vi "Potting Parameters.vi"(7 "Get/Set":enum16{"Get", "Set"}(ring), 8 "error in (no error)":errorcluster, 9 "Encapsulant":string, 10 "Potting Parameters in":T1, 11 "FlexWorktable in":refnum<class "FlexWorktable.lvclass">) -> (0 "error out":errorcluster, 2 "Potting Parameters out":T1, 3 "FlexWorktable out":refnum<class "FlexWorktable.lvclass">)   [LabVIEW 2017, in "FlexWorktable.lvclass"]
uses:
  FlexWorktable.lvclass
  Potting Parameters.ctl
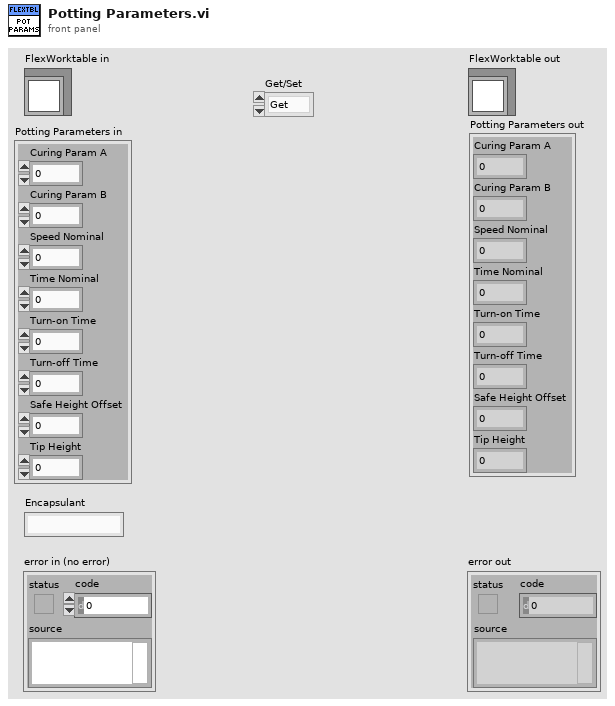
[diagram p1: front panel]
types:
  T1 = typedef "FlexWorktable.lvclass/Potting Parameters.ctl" = cluster{"Curing Param A":dbl, "Curing Param B":dbl, "Speed Nominal":dbl, "Time Nominal":dbl, "Turn-on Time":dbl, "Turn-off Time":dbl, "Safe Height Offset":dbl, "Tip Height":dbl}
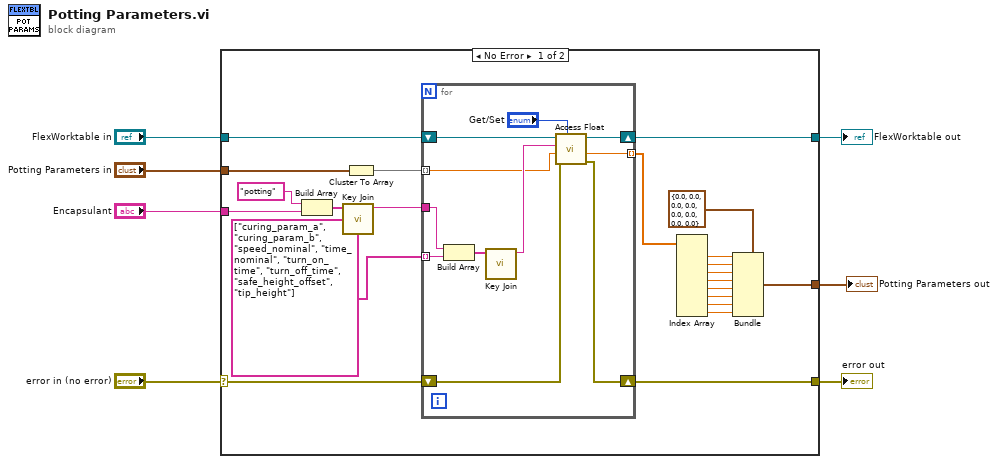
[diagram p0: block diagram]
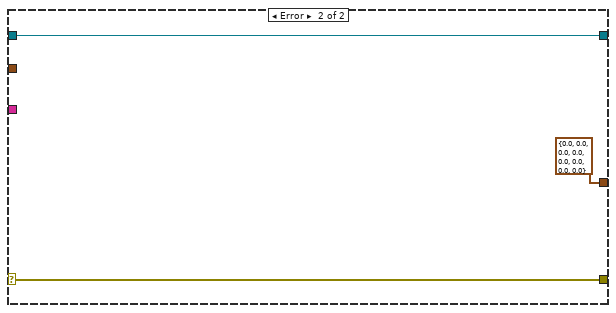
[diagram p2: hidden frame]
diagram:
  n1 = case shown="No Error" "error in (no error)" {
    selector: "error in (no error)" -> [w21 w43]
    tunnel: [w20 w43] -> w6
    tunnel: [w19 w42] -> w4
    tunnel: "FlexWorktable in" -> [w22 w42]
    tunnel: "Potting Parameters in" -> [w26 _]
    tunnel: "Encapsulant" -> [w27 _]
    tunnel: [w8 T1 {"Curing Param A"=0.0, "Curing Param B"=0.0, "Speed Nominal"=0.0, "Time Nominal"=0.0, "Turn-on Time"=0.0, "Turn-off Time"=0.0, "Safe Height Offset"=0.0, "Tip Height"=0.0} ("Potting Parameters in")] -> w1
    frame No Error {
      n2 = Build Array("potting", w27) -> (w29:string[])
      n3 = call "Key Join.vi"("Key Elements"=w29) -> ("Key"=w23:string)  [unwired: 10 in]
      n4 = Cluster To Array(cluster=w26) -> (array=w25:dbl[])
      n5 = for {
        tunnel: w25 -> [w34] mode=indexing
        tunnel: string[] ["curing_param_a", "curing_param_b", "speed_nominal", "time_nominal", "turn_on_time", "turn_off_time", "safe_height_offset", "tip_height"] -> [w39] mode=indexing
        tunnel: w23 -> [w40]
        shift-right: [w32] -> w20
        shift-left: w21 -> [w33]
        tunnel: [w31] -> w18 mode=indexing
        shift-right: [w30] -> w19
        shift-left: w22 -> [w35]
        n6 = Build Array(w40, w39) -> (w38:string[])
        n7 = call "Key Join.vi"("Key Elements"=w38) -> ("Key"=w37:string)  [unwired: 10 in]
        n8 = call-dynamic "Access Float.vi"("Get/Set"="Get/Set", "error in (no error)"=w33, "Value in"=w34, "Key"=w37, "FlexWorktable in"=w35) -> ("error out"=w32:errorcluster, "Value out"=w31:dbl, "FlexWorktable out"=w30:refnum<class "FlexWorktable.lvclass">)  [unwired: 4 in]
      }
      n9 = Index Array(array=w18) -> (element #1=w16:dbl, element #2=w15:dbl, element #3=w14:dbl, element #4=w13:dbl, element #5=w12:dbl, element #6=w11:dbl, element #7=w10:dbl, element #8=w9:dbl)  [unwired: 8 in]
      n10 = Bundle(cluster=T1 {"Curing Param A"=0.0, "Curing Param B"=0.0, "Speed Nominal"=0.0, "Time Nominal"=0.0, "Turn-on Time"=0.0, "Turn-off Time"=0.0, "Safe Height Offset"=0.0, "Tip Height"=0.0} ("Potting Parameters in"), "Curing Param A"=w16, "Curing Param B"=w15, "Speed Nominal"=w14, "Time Nominal"=w13, "Turn-on Time"=w12, "Turn-off Time"=w11, "Safe Height Offset"=w10, "Tip Height"=w9) -> (w8:T1)
    }
    frame Error {
    }
  }
  "error out" <- w6
  "FlexWorktable out" <- w4
  "Potting Parameters out" <- w1
